vi "Insert Parallel.vi"(8 "error in (no error)":errorcluster, 10 "Insert Parallel":T1, 11 "Test Executive Builder Model in":refnum<class "Test Executive Builder Model.lvclass">) -> (0 "error out":errorcluster, 3 "Test Executive Builder Model out":refnum<class "Test Executive Builder Model.lvclass">, 5 "Unique ID out":string)   [LabVIEW 2017, in "Test Executive Builder Model.lvclass"]
uses:
  Test Executive Builder Model.lvclass
  C:/Program Files/National Instruments/LabVIEW 2017/vi.lib/ActorFramework/Actor/Actor.lvclass
  Application Dependencies/Insert Parallel.ctl
  Test Executive Builder Model.lvclass/Test Executive Builder Model.ctl
  <vilib>/ActorFramework/Actor/Actor.lvclass/Actor.ctl
  <vilib>/ActorFramework/Message Enqueuer/Message Enqueuer.lvclass/Message Enqueuer.ctl
  <vilib>/ActorFramework/Message Enqueuer/Init from Existing Queue.vi
  <vilib>/ActorFramework/Message Enqueuer/Enqueue.vi
  Test Executive Builder Model Messages/Redraw Tree Msg/Redraw Tree Msg.lvclass
  C:/Program Files/National Instruments/LabVIEW 2017/vi.lib/ActorFramework/Message/Message.lvclass
  <vilib>/ActorFramework/Message Priority Queue/Priority Enqueue.vi
  <vilib>/ActorFramework/Message Enqueuer/Message Enqueuer.lvclass
  <vilib>/ActorFramework/Actor/Actor.lvclass
  <vilib>/gpm_packages/@cs/test-executive/Source/Test Executive/TestExecutive Ref/TestExecutive Ref.lvclass
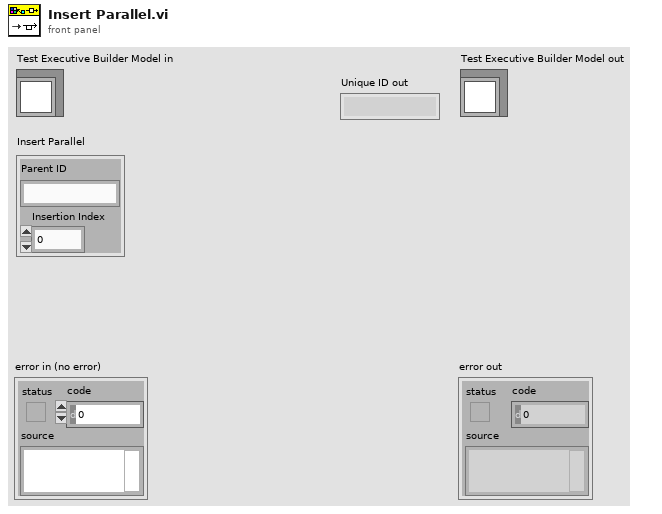
[diagram p1: front panel]
types:
  T1 = typedef "Insert Parallel.ctl" = cluster{"Parent ID":string, "Insertion Index":i32}
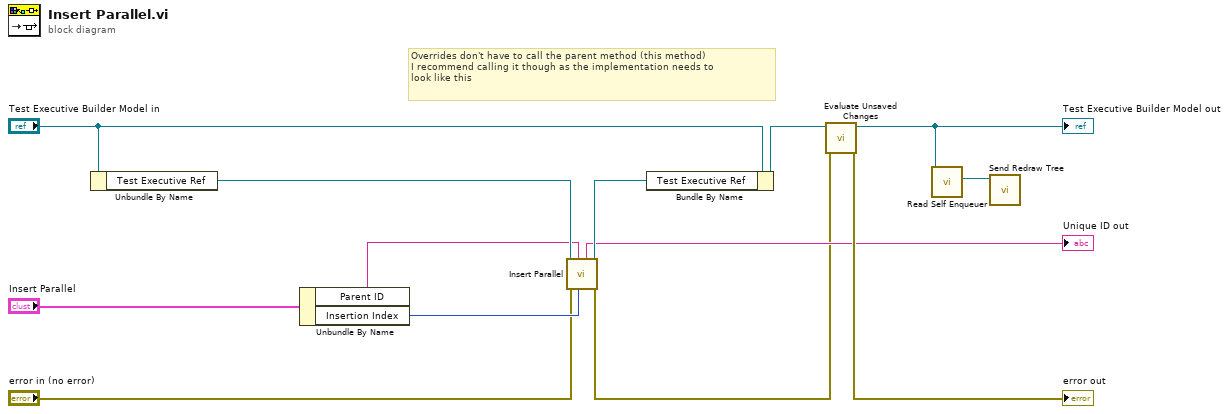
[diagram p0: block diagram]
diagram:
  # "Overrides don't have to call the parent method (this method)\nI recommend calling it though as the implementation needs to\nlook like this"
  n1 = Unbundle By Name("Test Executive Builder Model in") -> ("Test Executive Ref"=w8:refnum<data-value>)
  n2 = Unbundle By Name("Insert Parallel") -> ("Parent ID"=w6:string, "Insertion Index"=w3:i32)
  n3 = call <vilib>:"Insert Parallel.vi"("Insertion Index"=w3, "Parent ID"=w6, "error in (no error)"="error in (no error)", "Test Executive Ref"=w8) -> ("error out"=w4:errorcluster, "Test Executive Ref out"=w7:refnum<data-value>, "Unique ID out"=→"Unique ID out":string)  [unwired: 4 in, 1 out]
  n4 = Bundle By Name(cluster="Test Executive Builder Model in", "Test Executive Ref"=w7) -> (w11:refnum<class "Test Executive Builder Model.lvclass">)
  n5 = call-dynamic "Evaluate Unsaved Changes.vi"("error in (no error)"=w4, "Test Executive Builder Model in"=w11) -> ("error out"=→"error out":errorcluster, "Test Executive Builder Model out"=w10:refnum<class "Test Executive Builder Model.lvclass">)  [unwired: 8 in]
  "Test Executive Builder Model out" <- w10
  n6 = call <vilib>:"Read Self Enqueuer.vi"("Actor"=w10) -> ("Self Enqueuer"=w12:refnum<class "Message Enqueuer.lvclass">)  [unwired: 10 in]
  n7 = call "Send Redraw Tree.vi"("Message Enqueuer"=w12) -> ()  [unwired: 9 in, 2 out]
